vi "Core Action.vi"(8 "error in (no error)":errorcluster, 10 "SECS-II Class":refnum<class "SECS-II Class.lvclass">, 11 "Host Requests Status Variable Namelist in":refnum<class "02-Host Requests Status Variable Namelist.lvclass">) -> (0 "error out":errorcluster, 2 "SECS-II Class Out":refnum<class "SECS-II Class.lvclass">, 3 "Host Requests Status Variable Namelist out":refnum<class "02-Host Requests Status Variable Namelist.lvclass">)   [LabVIEW 2020, in "SECS Scenarios.lvlib" / "02-Host Requests Status Variable Namelist.lvclass"]
uses:
  02-Host Requests Status Variable Namelist.lvclass
  D:/Dropbox/SECS/SECS_GEM v1.1.0/Com/SECS Scenarios/Scenarios Class/Scenarios Class.lvclass
  SECS Communication/SECS-II Class/SECS-II Class.lvclass
  SECS Communication/S1 Message Class/S1 Message Class.lvclass
  D:/Dropbox/SECS/SECS_GEM v1.1.0/Com/SECS Communication/SECS-II Class/SECS-II Class.lvclass
  Scenarios Class/Scenarios Class.lvclass/Scenarios Class.ctl
  Scenarios Class/Reply State.ctl
  Scenarios Class/Write Reply State.vi
  Scenarios Class/Read HSMS Class.vi
  SECS Communication/SECS Data Class/Get SVID Data.vi
  SECS Communication/SECS Data Class/Get All SVID Data.vi
  SECS Communication/HSMS Class/HSMS Class.lvclass
  02-Host Requests Status Variable Namelist.lvclass/02-Host Requests Status Variable Namelist.ctl
  SECS Communication/SECS Data Class/SECS Data Class.lvclass
  Scenarios Class/Scenarios Class.lvclass
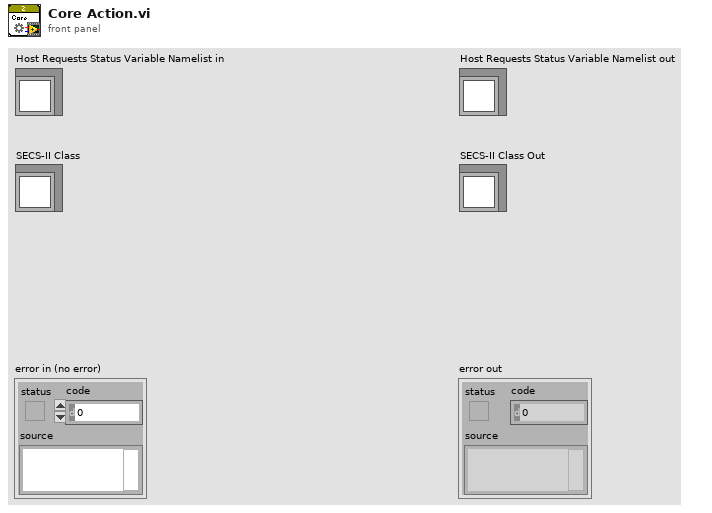
[diagram p1: front panel]
types:
  T1 = typedef "SECS Scenarios.lvlib/Scenarios Class.lvclass/Reply State.ctl" = enum16{"OK", "Illegal Data", "Unknown Stream", "Unknown Function", "Off-Line", "T3 Timeout", "Inner-Timeout"}
  T2 = cluster{"SVID":u32, "SVNAME":string, "UNITS":string}
  T3 = typedef "SECS Communication.lvlib/SECS Data Class.lvclass/SVID Data.ctl" = cluster{"SVID":u32, "Name":string, "Description":string, "Format Code":T4, "Unit":string, "Source":string, "Data":variant}
  T4 = typedef "SECS Communication.lvlib/SECS-II Class.lvclass/Format Code.ctl" = enum16{"L", "A", "B", "Boolean", "J", "I1", "I2", "I4", "I8", "U1", "U2", "U4", "U8", "F4", "F8", "Char"}
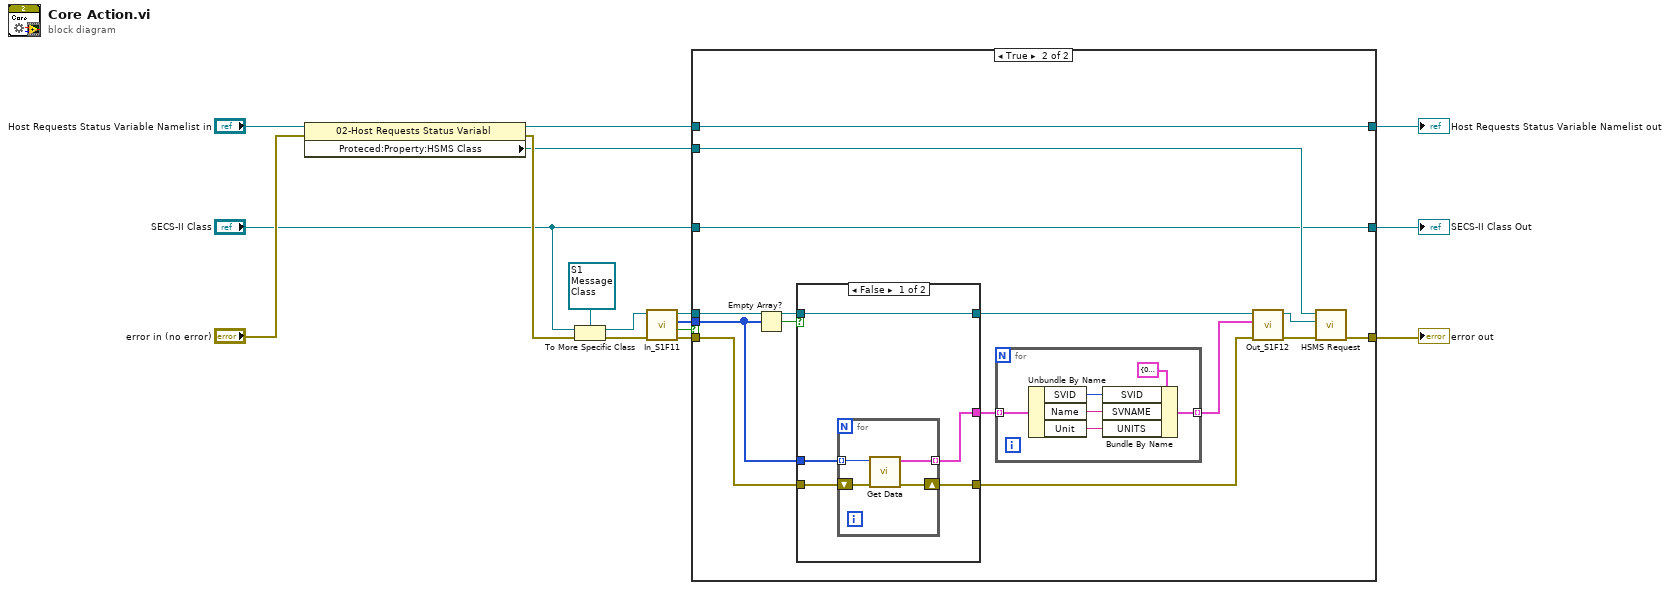
[diagram p0: block diagram]
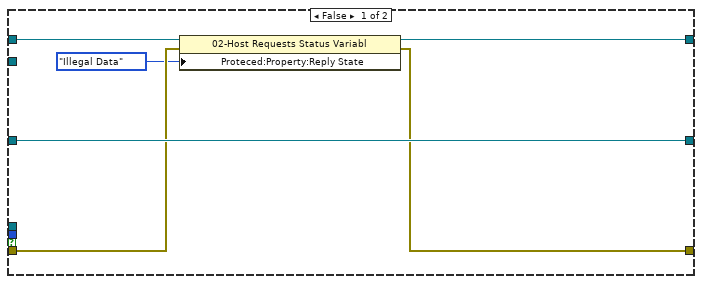
[diagram p2: hidden frame]
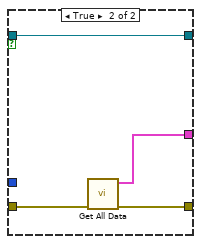
[diagram p3: hidden frame]
diagram:
  n1 = property class="02-Host Requests Status Variabl"(reference="Host Requests Status Variable Namelist in", error in="error in (no error)") -> (reference out=w2:refnum<class "02-Host Requests Status Variable Namelist.lvclass">, error out=w14:errorcluster, "Proteced:Property:HSMS Class"=w10:refnum<class "HSMS Class.lvclass">)
  n2 = To More Specific Class(target class=refnum<class "S1 Message Class.lvclass"> refnum ("S1 Message Class in"), reference="SECS-II Class", error in=w14) -> (specific class reference=w12:refnum<class "S1 Message Class.lvclass">, error out=w13:errorcluster)
  n3 = call "In_S1F11.vi"("error in (no error)"=w13, "S1 Message Class in"=w12) -> ("error out"=w11:errorcluster, "OK?"=w5:bool, "Status Variable ID(SVID)"=w8:u32[], "S1 Message Class out"=w7:refnum<class "S1 Message Class.lvclass">)  [unwired: 6 in]
  n4 = case shown="True" w5 {
    tunnel: w11 -> [w19 w36]
    tunnel: w10 -> [_ w33]
    tunnel: [w18 w32] -> w9
    tunnel: w8 -> [_ w28]
    tunnel: w7 -> [_ w26]
    tunnel: "SECS-II Class" -> [w20 w24]
    tunnel: [w20 w24] -> w3
    tunnel: w2 -> [w22 w23]
    tunnel: [w21 w23] -> w1
    frame False {
      n5 = property class="02-Host Requests Status Variabl"(reference=w22, error in=w19, "Proteced:Property:Reply State"=Reply_State."Illegal Data" ("Reply State")) -> (reference out=w21:refnum<class "02-Host Requests Status Variable Namelist.lvclass">, error out=w18:errorcluster)
    }
    frame True {
      n6 = Empty Array?(array=w28) -> (empty?=w27:bool)
      n7 = case shown="False" w27 {
        tunnel: w36 -> [w41 w49]
        tunnel: [w40 w47] -> w31
        tunnel: [w39 w48] -> w29
        tunnel: w28 -> [w38 _]
        tunnel: w26 -> [w37 w46]
        tunnel: [w37 w46] -> w25
        frame False {
          n8 = for {
            tunnel: w38 -> [w44] mode=indexing
            shift-right: [w43] -> w39
            shift-left: w41 -> [w45]
            tunnel: [w42] -> w40 mode=indexing
            n9 = call-poly "Get Data.vi"("error in"=w45, "SVID"=w44) -> ("error out"=w43:errorcluster, "SVID Data"=w42:T3)  [unwired: 7 in, 1 out]
          }
        }
        frame True {
          n10 = call-poly "Get All Data.vi"("error in (no error)"=w49) -> ("error out"=w48:errorcluster, "SVID Data"=w47:T3[])  [unwired: 9 in]
        }
      }
      n11 = for {
        tunnel: w31 -> [w54] mode=indexing
        tunnel: [w50] -> w30 mode=indexing
        n12 = Unbundle By Name(w54) -> ("SVID"=w53:u32, "Name"=w52:string, "Unit"=w51:string)
        n13 = Bundle By Name(cluster=T2 {"SVID"=0, "SVNAME"="", "UNITS"=""} ("S1F12"), "SVID"=w53, "SVNAME"=w52, "UNITS"=w51) -> (w50:T2)
      }
      n14 = call "Out_S1F12.vi"("error in (no error)"=w29, "S1F12"=w30, "S1 Message Class in"=w25) -> ("error out"=w35:errorcluster, "S1 Message Class out"=w34:refnum<class "S1 Message Class.lvclass">)  [unwired: 7 in]
      n15 = call "HSMS Request.vi"("error in (no error)"=w35, "SECS-II Class In"=w34, "HSMS Class in"=w33) -> ("error out"=w32:errorcluster)  [unwired: 7 in, 1 out]
    }
  }
  "error out" <- w9
  "Host Requests Status Variable Namelist out" <- w1
  "SECS-II Class Out" <- w3
